vi "Launch Turbo.vi"(8 "error in (no error)":errorcluster, 11 "cRIO-CO2 in":refnum<class "cRIO-CO2.lvclass">) -> (0 "error out":errorcluster, 3 "cRIO-CO2 out":refnum<class "cRIO-CO2.lvclass">)   [LabVIEW 2015, in "cRIO-Carbondioxide.lvlib" / "cRIO-CO2.lvlib" / "cRIO-CO2.lvclass"]
uses:
  cRIO-CO2.lvclass
  Turbo/Turbo.lvclass
  CO2 Actor/CO2 Actor.lvclass
  <vilib>/ActorFramework/Actor/Actor.lvclass
  cRIO-CO2.lvclass/cRIO-CO2.ctl
  cRIO-CO2 Messages/Log Message Msg/Log Message Msg.lvclass/Log Message Msg.ctl
  <vilib>/ActorFramework/Message Enqueuer/Message Enqueuer.lvclass/Message Enqueuer.ctl
  <vilib>/ActorFramework/Message Enqueuer/Enqueue.vi
  <vilib>/ActorFramework/Message Priority Queue/Priority Enqueue.vi
  <vilib>/ActorFramework/Message Enqueuer/Message Enqueuer.lvclass
  cRIO-CO2 Messages/Log Message Msg/Log Message Msg.lvclass
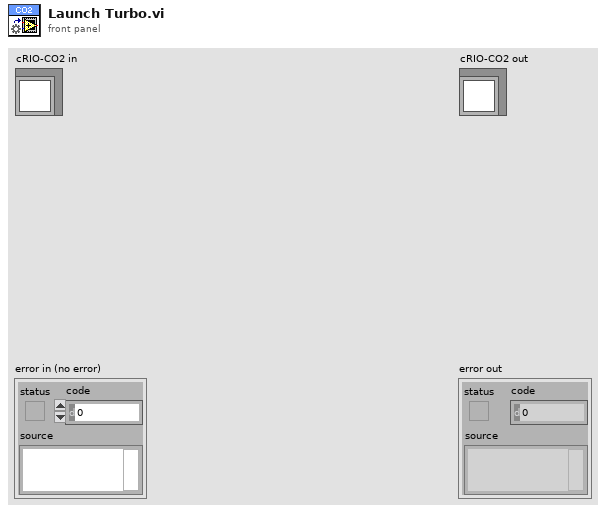
[diagram p1: front panel]
types:
  T1 = typedef "Dedicated Enqueuers.ctl" = cluster{"Freezers":cluster{"Syringe":refnum<class "Message Enqueuer.lvclass">, "Tank 1":refnum<class "Message Enqueuer.lvclass">, "Tank 2":refnum<class "Message Enqueuer.lvclass">, "Tank 3":refnum<class "Message Enqueuer.lvclass">, "Tank 4":refnum<class "Message Enqueuer.lvclass">}, "Heaters":cluster{"Syringe":refnum<class "Message Enqueuer.lvclass">, "Piston":refnum<class "Message Enqueuer.lvclass">}, "Blowers":cluster{"Tank 1":refnum<class "Message Enqueuer.lvclass">, "Tank 2":refnum<class "Message Enqueuer.lvclass">, "Tank 3":refnum<class "Message Enqueuer.lvclass">, "Tank 4":refnum<class "Message Enqueuer.lvclass">, "Syringe":refnum<class "Message Enqueuer.lvclass">}, "Sample Line":refnum<class "Message Enqueuer.lvclass">, "Storage Line":refnum<class "Message Enqueuer.lvclass">, "Transfer Line":refnum<class "Message Enqueuer.lvclass">, "Syringe Stepper":refnum<class "Message Enqueuer.lvclass">, "Syringe Line":refnum<class "Message Enqueuer.lvclass">, "Capillary Line":refnum<class "Message Enqueuer.lvclass">, "Preparation Line":refnum<class "Message Enqueuer.lvclass">, "Turbo":refnum<class "Message Enqueuer.lvclass">, "Vacuum":refnum<class "Message Enqueuer.lvclass">, "He Line":refnum<class "Message Enqueuer.lvclass">, "Cylinder":refnum<class "Message Enqueuer.lvclass">}
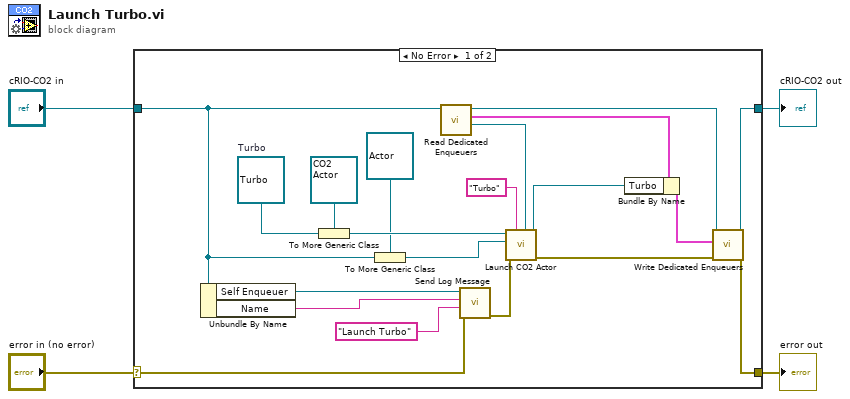
[diagram p0: block diagram]
diagram:
  n1 = case shown="No Error" "error in (no error)" {
    selector: "error in (no error)" -> [w21 w26]
    tunnel: [w14 w26] -> w3
    tunnel: [w15 w25] -> w1
    tunnel: "cRIO-CO2 in" -> [w12 w25]
    frame No Error {
      w24 = refnum<class "Turbo.lvclass"> refnum  # Turbo
      n2 = Unbundle By Name(w12) -> ("Self Enqueuer"=w13:refnum<class "Message Enqueuer.lvclass">, "Name"=w19:string)
      n3 = To More Generic Class(target class=refnum<class "CO2 Actor.lvclass"> refnum ("CO2 Actor in"), reference=w24) -> (generic class reference=w23:refnum<class "CO2 Actor.lvclass">)
      n4 = To More Generic Class(target class=refnum<class "Actor.lvclass"> refnum ("Caller Actor in"), reference=w12) -> (generic class reference=w10:refnum<class "Actor.lvclass">)
      n5 = call "Read Dedicated Enqueuers.vi"("cRIO-CO2 in"=w12) -> ("Qs.DedicatedEnQrs"=w8:refnum<queue>, "Dedicated Enqueuers"=w6:T1, "cRIO-CO2 out"=w7:refnum<class "cRIO-CO2.lvclass">)  [unwired: 7 in, 1 out]
      n6 = call "Send Log Message.vi"("error in (no error)"=w21, "String"="Launch Turbo", "Source Name"=w19, "Message Enqueuer"=w13) -> ("error out"=w20:errorcluster)  [unwired: 6 in, 1 out]
      n7 = call "Launch CO2 Actor.vi"("DedicatedEnQrs"=w8, "Name"="Turbo", "error in (no error)"=w20, "Caller Actor in"=w10, "CO2 Actor in"=w23) -> ("error out"=w5:errorcluster, "Caller-To-Actor Enqueuer"=w17:refnum<class "Message Enqueuer.lvclass">)  [unwired: 5 in]
      n8 = Bundle By Name(cluster=w6, "Turbo"=w17) -> (w16:T1)
      n9 = call "Write Dedicated Enqueuers.vi"("error in (no error)"=w5, "Dedicated Enqueuers"=w16, "cRIO-CO2 in"=w7) -> ("error out"=w14:errorcluster, "cRIO-CO2 out"=w15:refnum<class "cRIO-CO2.lvclass">)  [unwired: 7 in]
    }
    frame Error {
    }
  }
  "error out" <- w3
  "cRIO-CO2 out" <- w1
